vi "Write File.vi"(6 "operation":T1(ring)=enum."replace or create with confirmation", 8 "error in (no error)":errorcluster, 9 "Data":variant, 10 "datalog path (use dialog)":path, 11 "Section File Interface":refnum<class "Section File Interface.lvclass">) -> (0 "error out":errorcluster)   [LabVIEW 2020, in "ImportExport.lvlib" / "Section File Interface.lvclass"]
uses:
  Section File Interface.lvclass
  <vilib>/NI/NI VeriStand Advanced SysDef API/_Types/File.DataType.ctl
  <vilib>/NI/NI VeriStand Advanced SysDef API/_SubVIs/SysDef.Globals.vi
  <vilib>/NI/NI VeriStand Advanced SysDef API/SysDef API/Advanced System Definition.lvlib
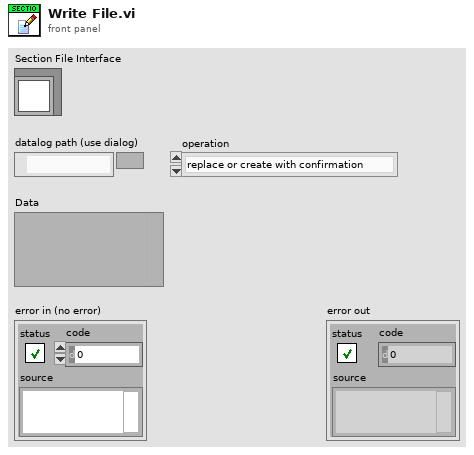
[diagram p1: front panel]
types:
  T1 = enum16{"open", "replace", "create", "open or create", "replace or create", "replace or create with confirmation"}
  T2 = typedef "Advanced System Definition.lvlib/File.DataType.ctl" = cluster{"Version":string, "Data":variant}
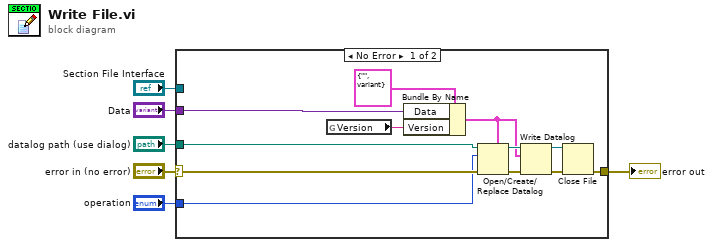
[diagram p0: block diagram]
diagram:
  n1 = case shown="No Error" "error in (no error)" {
    selector: "error in (no error)" -> [w11 w19]
    tunnel: [w10 w19] -> w5
    tunnel: "Section File Interface" -> [_ _]
    tunnel: "Data" -> [w12 _]
    tunnel: "datalog path (use dialog)" -> [w9 _]
    tunnel: "operation" -> [w7 _]
    frame No Error {
      n2 = global read "SysDef.Globals.vi" "Version"() -> (w8:string)
      n3 = Bundle By Name(cluster=T2 {"Version"="", "Data"=variant}, "Data"=w12, "Version"=w8) -> (w15:T2)
      n4 = Open/Create/Replace Datalog(5:w15, 8:w11, 10:w7, 11:w9) -> (0:w17:errorcluster, 3:w16:refnum<k1>)  [unwired: 2 in, 1 out]
      n5 = Write Datalog(4:w17, 6:w15, 7:w16) -> (0:w14:errorcluster, 3:w13:refnum<k1>)
      n6 = Close File(refnum=w13, error in=w14) -> (error out=w10:errorcluster)  [unwired: 1 out]
    }
    frame Error {
    }
  }
  "error out" <- w5
